vi "Insert Views.vi"(8 "error in (no error)":errorcluster, 10 "Full Factory in":refnum<class "Full Factory.lvclass">, 11 "UI Controller in":refnum<class "UI Controller.lvclass">) -> (0 "error out":errorcluster, 3 "UI Controller out":refnum<class "UI Controller.lvclass">)   [LabVIEW 2020, in "UI Controller.lvlib" / "Full Factory.lvclass"]
uses:
  Full Factory.lvclass
  UI Controller/UI Controller.lvclass
panel:
  # "NOTICE -- YOU MUST LEAVE THIS NOTICE IN PLACE.\n\nCopyright (c) 2017, LIANG LIU Shawn.Liu.cn@gmail.com\nAll rights reserved.\n\nRedistribution and use in source and binary forms, with or without modification, are permitted provided that the following conditions are met:\n-Redistributions of source code must retain the above copyright notice, this list of conditions and the following disclaimer.\n-Redistributions in binary form must reproduce the above copyright notice, this list of conditions and the following disclaimer in the documentation and/or other materials provided with the distribution.\n-Neither the name of the eLp nor the names of its contributors may be used to endorse or promote products derived from this software without specific prior written permission.\n\nTHIS SOFTWARE IS PROVIDED BY THE COPYRIGHT HOLDERS AND CONTRIBUTORS \"AS IS\" AND ANY EXPRESS OR IMPLIED WARRANTIES, INCLUDING, BUT NOT LIMITED TO, THE IMPLIED WARRANTIES OF MERCHANTABILITY AND FITNESS FOR A PARTICULAR PURPOSE ARE DISCLAIMED. IN NO EVENT SHALL THE COPYRIGHT HOLDER OR CONTRIBUTORS BE LIABLE FOR ANY DIRECT, INDIRECT, INCIDENTAL, SPECIAL, EXEMPLARY, OR CONSEQUENTIAL DAMAGES (INCLUDING, BUT NOT LIMITED TO, PROCUREMENT OF SUBSTITUTE GOODS OR SERVICES; LOSS OF USE, DATA, OR PROFITS; OR BUSINESS INTERRUPTION) HOWEVER CAUSED AND ON ANY THEORY OF LIABILITY, WHETHER IN CONTRACT, STRICT LIABILITY, OR TORT (INCLUDING NEGLIGENCE OR OTHERWISE) ARISING IN ANY WAY OUT OF THE USE OF THIS SOFTWARE, EVEN IF ADVISED OF THE POSSIBILITY OF SUCH DAMAGE."
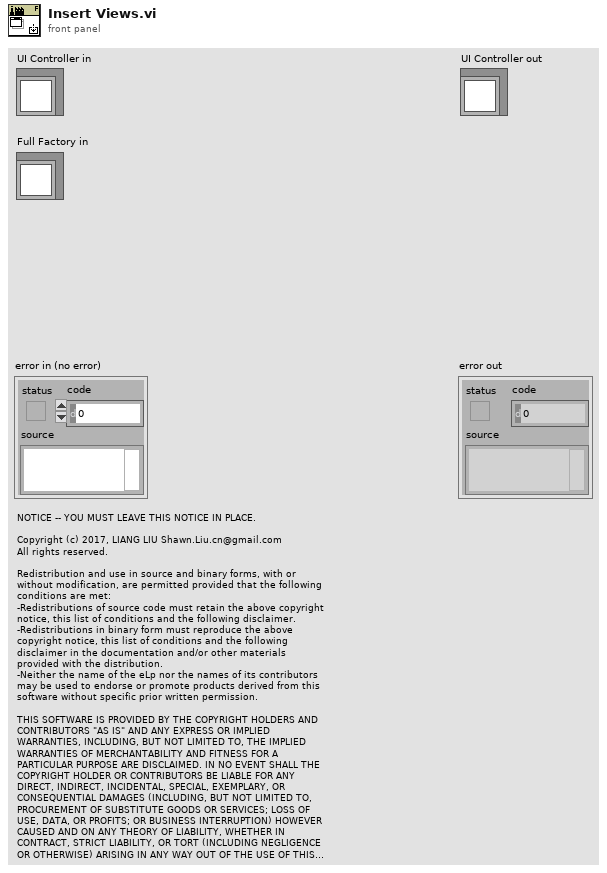
[diagram p1: front panel]
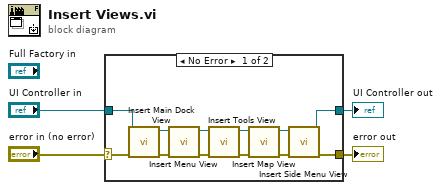
[diagram p0: block diagram]
diagram:
  n1 = case shown="No Error" "error in (no error)" {
    selector: "error in (no error)" -> [w8 w18]
    tunnel: [w7 w18] -> w3
    tunnel: "UI Controller in" -> [w6 w17]
    tunnel: [w5 w17] -> w1
    frame No Error {
      n2 = call "Insert Main Dock View.vi"("error in (no error)"=w8, "UI Controller in"=w6) -> ("error out"=w15:errorcluster, "UI Controller out"=w16:refnum<class "UI Controller.lvclass">)  [unwired: 8 in]
      n3 = call "Insert Menu View.vi"("error in (no error)"=w15, "UI Controller in"=w16) -> ("error out"=w13:errorcluster, "UI Controller out"=w14:refnum<class "UI Controller.lvclass">)  [unwired: 8 in]
      n4 = call "Insert Tools View.vi"("error in (no error)"=w13, "UI Controller in"=w14) -> ("error out"=w11:errorcluster, "UI Controller out"=w12:refnum<class "UI Controller.lvclass">)  [unwired: 8 in]
      n5 = call "Insert Map View.vi"("error in (no error)"=w11, "UI Controller in"=w12) -> ("error out"=w9:errorcluster, "UI Controller out"=w10:refnum<class "UI Controller.lvclass">)  [unwired: 8 in]
      n6 = call "Insert Side Menu View.vi"("error in (no error)"=w9, "UI Controller in"=w10) -> ("error out"=w7:errorcluster, "UI Controller out"=w5:refnum<class "UI Controller.lvclass">)  [unwired: 8 in]
    }
    frame Error {
    }
  }
  "error out" <- w3
  "UI Controller out" <- w1
